vi "Read Name Specs.vi"(11 "_Rename in":refnum<class "_Rename.lvclass">) -> (2 "Name Specs":refnum<class "Name Specs.lvclass">)   [LabVIEW 2025, in "_Rename.lvlib" / "_Rename.lvclass"]
uses:
  _Rename.lvclass
  _Rename.lvclass/_Rename.ctl
  _Shared/Name Specs/Name Specs.lvclass
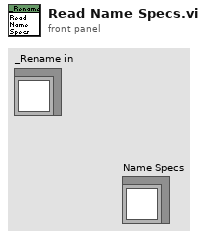
[diagram p1: front panel]
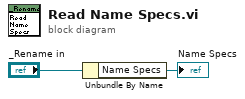
[diagram p0: block diagram]
diagram:
  n1 = Unbundle By Name("_Rename in") -> ("Name Specs"=→"Name Specs":refnum<class "Name Specs.lvclass">)
